vi "readFromXML.vi"(8 "error in (no error)":errorcluster, 10 "XML in":string, 11 "Difftrack in":refnum<class "Difftrack.lvclass">) -> (0 "error out":errorcluster, 3 "Difftrack out":refnum<class "Difftrack.lvclass">)   [LabVIEW 2014, in "TCSDataDefinitions.lvlib" / "TCSCommand.lvlib" / "TargetConfiguration.lvlib" / "Target.lvlib" / "Difftrack.lvclass"]
uses:
  Difftrack.lvclass
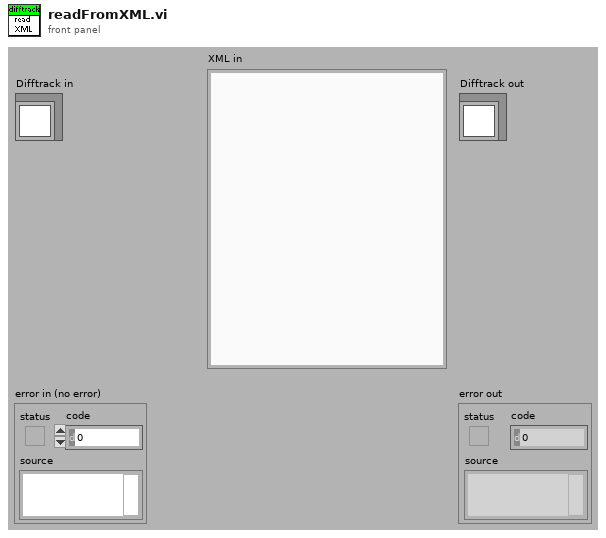
[diagram p1: front panel]
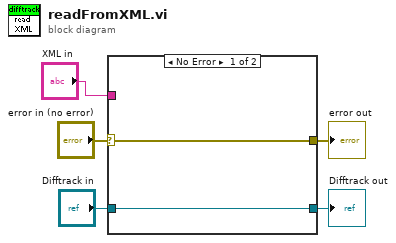
[diagram p0: block diagram]
diagram:
  n1 = case shown="No Error" "error in (no error)" {
    selector: "error in (no error)" -> [w6 w9]
    tunnel: [w6 w9] -> w4
    tunnel: [w7 w8] -> w2
    tunnel: "Difftrack in" -> [w7 w8]
    tunnel: "XML in" -> [_ _]
    frame No Error {
    }
    frame Error {
    }
  }
  "error out" <- w4
  "Difftrack out" <- w2
